vi "Get Malleable VI Name.vi"(8 "error in (no error)":errorcluster, 11 "SubVI Ref In":refnum<vi>) -> (0 "error out":errorcluster, 1 "Name without extension":string, 2 "Is Malleable VI?":bool, 3 "SubVI Ref Out":refnum<vi>, 4 "Name (unmodified)":string)   [LabVIEW 2020]
doc: "Determines if the subVI reference is to a malleable VI instance, and returns the name of the malleable VI."
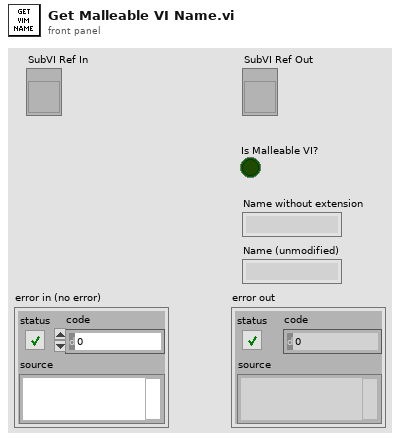
[diagram p1: front panel]
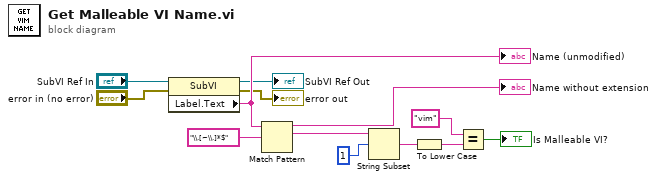
[diagram p0: block diagram]
diagram:
  n1 = property class="SubVI"(reference="SubVI Ref In", error in="error in (no error)") -> (reference out=→"SubVI Ref Out":refnum<vi>, error out=→"error out":errorcluster, "Label.Text"=w12:string)
  "Name (unmodified)" <- w12
  n2 = Match Pattern(string=w12, regular expression="\\.[~\\.]*$") -> (before substring=→"Name without extension":string, match substring=w8:string)  [unwired: 3 out]
  n3 = String Subset(string=w8, offset (0)=1) -> (substring=w7:string)  [unwired: 1 out]
  n4 = To Lower Case(string=w7) -> (all lower case string=w11:string)
  n5 = Equal?(x="vim", y=w11) -> (x = y?=→"Is Malleable VI?":bool)
